vi "Create RSA CNG Algorithm.vi"(8 "error in (no error)":errorcluster) -> (0 "error out":errorcluster, 3 "RSA Cng Algorithm":refnum<k24>)   [LabVIEW 2021, in "dotNET Crypto Key Management.lvlib"]
doc: "Generates an instance of a .NET CNG Algorithm object for the RSA algorithm."
uses:
  dotNET Crypto Key Management.lvlib
  System.Core
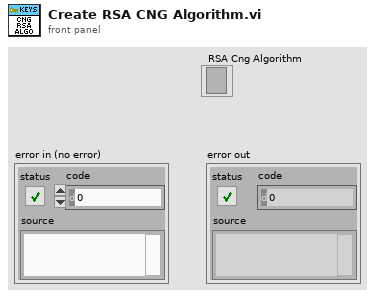
[diagram p1: front panel]
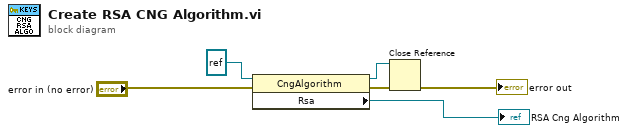
[diagram p0: block diagram]
diagram:
  n1 = property class="CngAlgorithm"(reference=refnum<k24> refnum ("algorithm"), error in="error in (no error)") -> (reference out=w6:refnum<k24>, error out=w1:errorcluster, "Rsa"=→"RSA Cng Algorithm":refnum<k24>)
  n2 = Close Reference(reference=w6, error in (no error)=w1) -> (error out=→"error out":errorcluster)
